vi "HexToString.vi"(11 "数组":u16[](array[numeric]) format="%04xH") -> (3 "字符串":string)   [LabVIEW 2016, in "斯坦道CODMn.lvlib"]
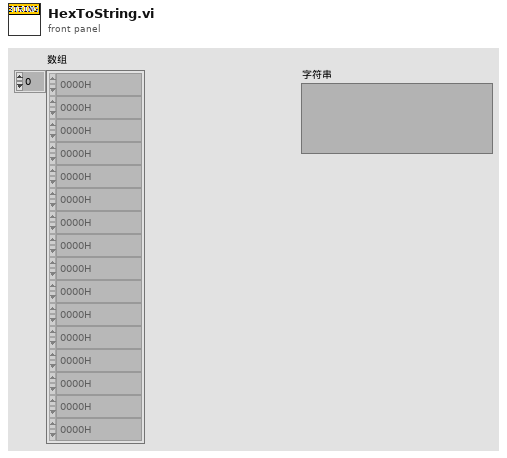
[diagram p1: front panel]
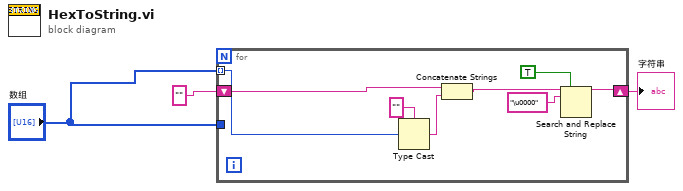
[diagram p0: block diagram]
diagram:
  n1 = for {
    tunnel: "数组" -> [w8] mode=indexing
    tunnel: "数组" -> [_]
    shift-right: [w4] -> w1
    shift-left: "" -> [w9]
    n2 = Type Cast(type="", x=w8) -> (*(type *) &x=w10:string)
    n3 = Concatenate Strings(w9, w10) -> (w5:string)
    n4 = Search and Replace String(replace all?=TRUE ("替换全部？(F)"), input string=w5, search string="\u0000" ("搜索字符串")) -> (result string=w4:string)  [unwired: 5 in, 3 out]
  }
  "字符串" <- w1
